vi "Add Address Write Info.vi"(9 "terminal handle":u64, 10 "terminal address":T1, 11 "address write info array":T2[](array[typedef])) -> (3 "address write info array out":T2[](array[typedef]))   [LabVIEW 2020, in "Ballard MIL-STD-1553 Engine.lvlib" / "Custom Device.lvlib"]
uses:
  Custom Device.lvlib
  Shared/Address.ctl
  Implementation/Address Based Execution Unit/Address Write Info.ctl
  Implementation/Address Based Execution Unit/Address Based Execution Unit.lvclass
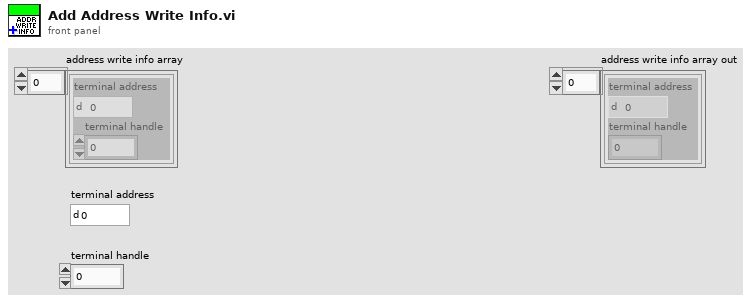
[diagram p1: front panel]
types:
  T1 = typedef "Address.ctl" = u16
  T2 = typedef "Ballard MIL-STD-1553 Engine.lvlib/Implementation.lvlib/Address Based Execution Unit.lvclass/Address Write Info.ctl" = cluster{"terminal address":T1, "terminal handle":u64}
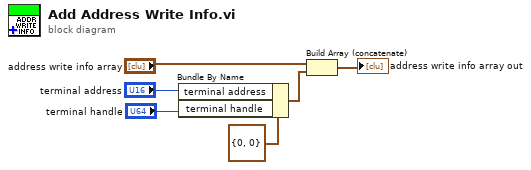
[diagram p0: block diagram]
diagram:
  n1 = Bundle By Name(cluster=T2 {"terminal address"=0, "terminal handle"=0} ("address write info"), "terminal address"="terminal address", "terminal handle"="terminal handle") -> (w6:T2)
  n2 = Build Array (concatenate)("address write info array", w6) -> (→"address write info array out":T2[])
